vi "Main.vi"() -> ()   [LabVIEW 2017]
doc: "The boiler controller allows a user to start and shut down a boiler.\nUse the Reset, start and Light pilot to sequencially Start the boiler.\nUse the fuel control valve to change the flow of fulel into the boiler.\nUse the Stop button to Shut down the boiler.\nTo shut down the system off ar in the event of emergency, use the emergency stop button to stop the application completely."
uses:
  controls/MHL Data.ctl
  controls/MHL UI Data.ctl
  controls/MHL Status.ctl
  controls/MHL References.ctl
  controls/MHL Configuration.ctl
  support/Boiler System Globals.vi
  <vilib>/Utility/error.llb/Error Cluster From Error Code.vi
  <vilib>/ErrorRing/Error Ring.xnode
  support/Message Queue/Message Queue.lvlib
  support/User Event - Stop/User Event - Stop.lvlib
  Controller/Controller.lvlib
  Boiler/Boiler.lvlib
panel:
  out "Forced Draft Fan":bool
  out "Pilot LED":bool caption="Pilot"
  out "Pilot Gas Valve":bool
  out "Primany Fan":bool
  in  "Fuel Control Valve":u32(slide) scale=10.0..75.0
  in  "Initiate Stop":bool
  in  "Shutdown":bool
  in  "Pilot":bool
  in  "Start Sequence":bool
  in  "Reset":bool
  out "Status":string
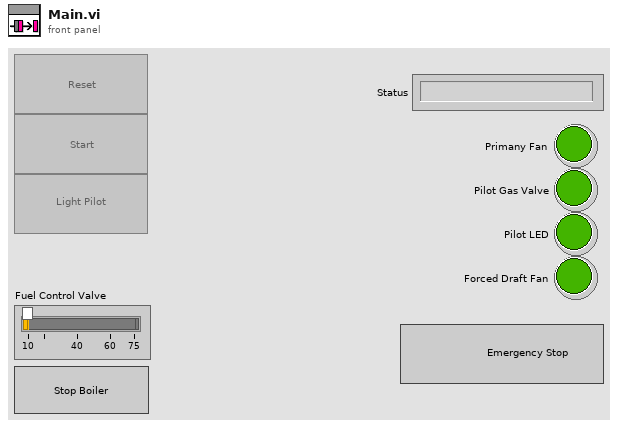
[diagram p1: front panel]
types:
  T1 = typedef "MHL Data.ctl" = cluster{"MHL User Interface Data":T2, "MHL References":T4, "MHL Configuration":T5}
  T2 = typedef "MHL UI Data.ctl" = cluster{"Status":string, "Fuel Control Valve":u32, "Primary Fan":bool, "Pilot Gas Valve":bool, "Pilot":bool, "Forced Draft Fan":bool, "MHL Status":T3}
  T3 = typedef "MHL Status.ctl" = enum16{"Lockout", "Ready", "Pre-Purge", "Pre-Purge Complete", "Pilot On", "Boiler Running", "Shutdown", "Purge"}
  T4 = typedef "MHL References.ctl" = cluster{"Reset Ref":refnum<vi>, "Start Sequence Ref":refnum<vi>, "Pilot Ref":refnum<vi>, "Shutdown Ref":refnum<vi>, "Fuel Control Valve Ref":refnum<vi>}
  T5 = typedef "MHL Configuration.ctl" = cluster{"Fuel Control Valve Maximum":dbl, "Fuel Control Valve Minimum":dbl}
  T6 = typedef "Configuration Data.ctl" = cluster{"MHL Configuration":T5, "Controller Configuration":T7, "Boiler Configuration":T8}
  T7 = typedef "Controller.lvlib/Controller Configuration.ctl" = cluster{"Purge Time":u32, "Flame Threshold":u32}
  T8 = typedef "Boiler.lvlib/Boiler Configuration.ctl" = cluster{"Pilot Increment (ms)":u32, "Pilot Decrement (ms)":u32}
  T9 = typedef "Notifiers.ctl" = cluster{"Handshake":refnum<notifier>, "Flame Level":refnum<notifier>, "Controller Exit":refnum<notifier>, "Boiler Exit":refnum<notifier>}
  T10 = typedef "Message Queue.lvlib/All Message Queues.ctl" = cluster{"MHL":refnum<queue>, "Boiler Controller":refnum<queue>, "Boiler":refnum<queue>}
  T11 = enum16{"open", "replace", "create", "open or create", "replace or create", "replace or create with confirmation"}
  T12 = enum32{"invalid app kind", "Development System", "Run Time System", "Student Edition", "Embedded LabVIEW", "Evaluation", "Custom"}
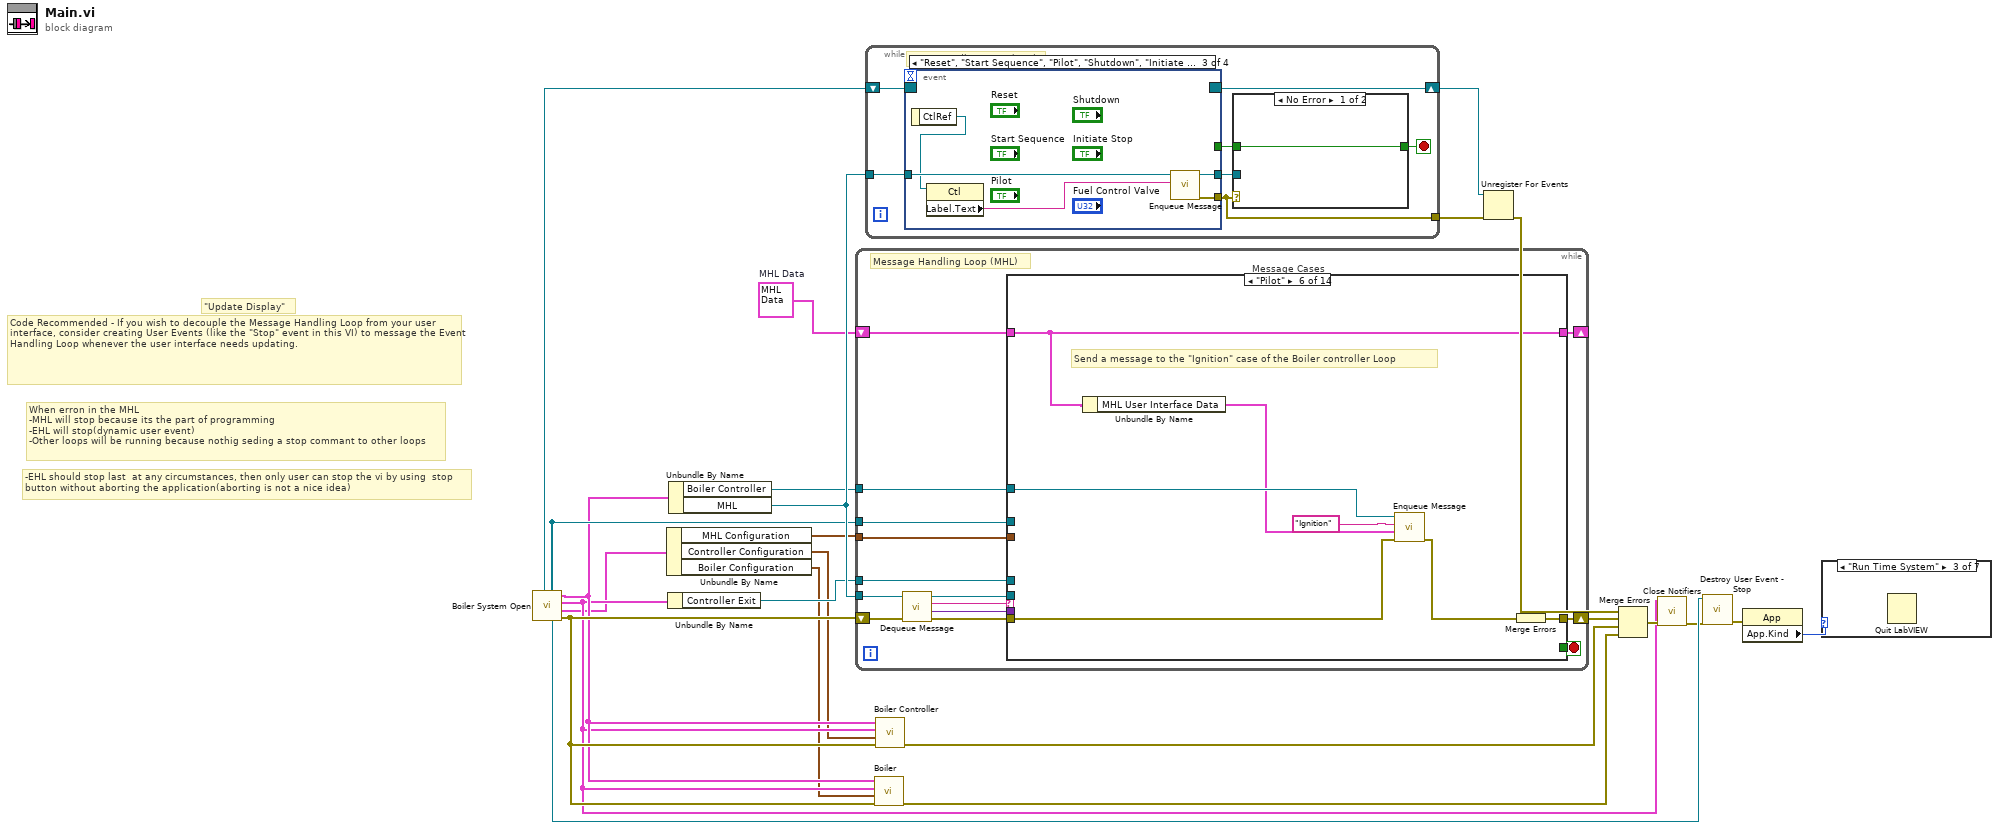
[diagram p0: block diagram]
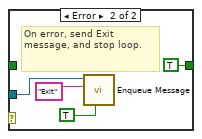
[diagram p8: hidden frame]
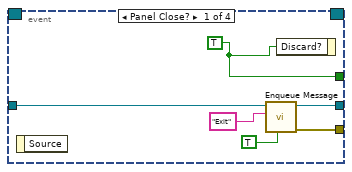
[diagram p9: hidden frame]
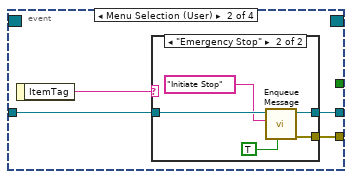
[diagram p10: hidden frame]
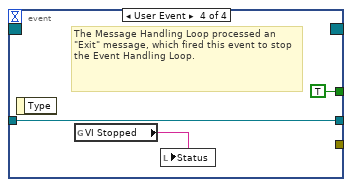
[diagram p12: hidden frame]
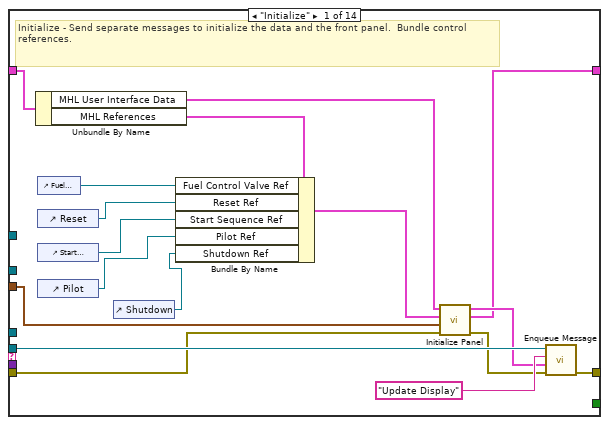
[diagram p13: hidden frame]
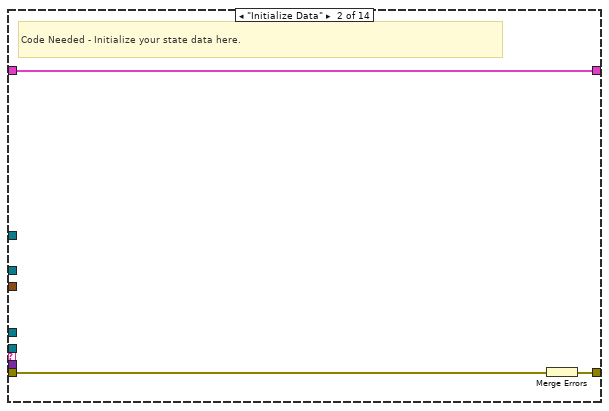
[diagram p14: hidden frame]
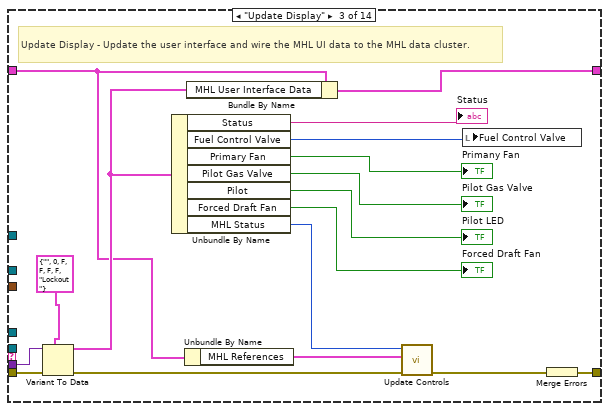
[diagram p15: hidden frame]
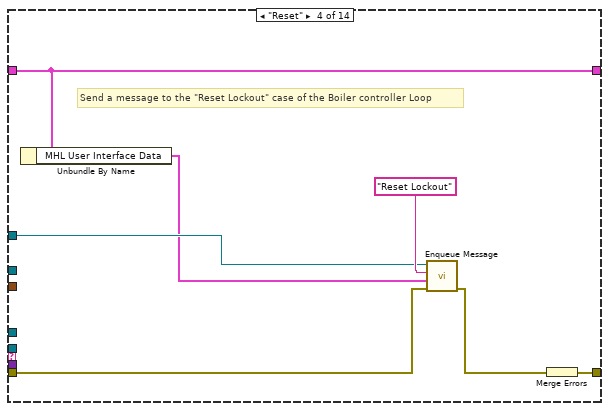
[diagram p16: hidden frame]
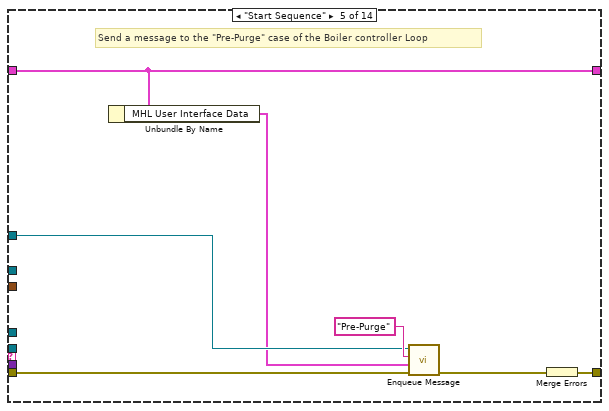
[diagram p17: hidden frame]
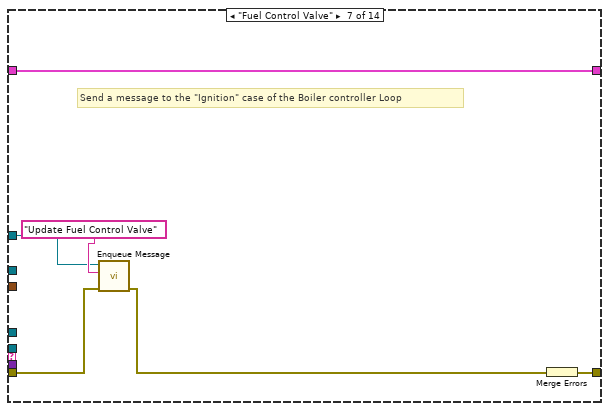
[diagram p18: hidden frame]
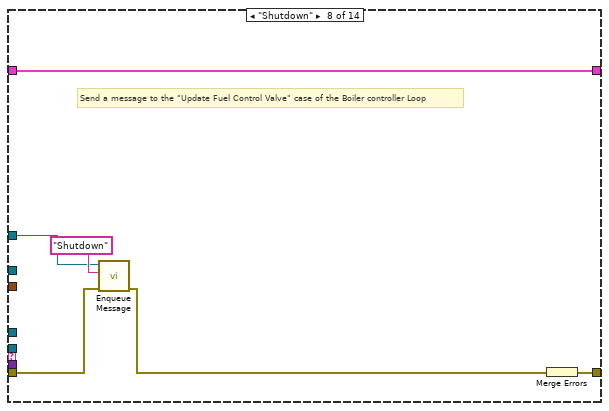
[diagram p19: hidden frame]
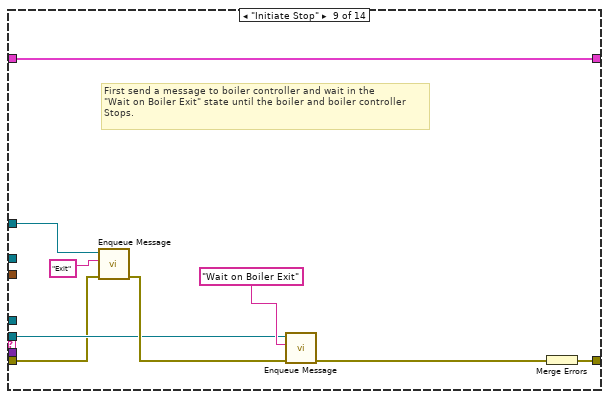
[diagram p20: hidden frame]
diagram:
  w9 = T1 {"MHL User Interface Data"={"Status"="", "Fuel Control Valve"=0, "Primary Fan"=FALSE, "Pilot Gas Valve"=FALSE, "Pilot"=FALSE, "Forced Draft Fan"=FALSE, "MHL Status"=enum."Lockout"}, "MHL References"={"Reset Ref"=refnum, "Start Sequence Ref"=refnum, "Pilot Ref"=refnum, "Shutdown Ref"=refnum, "Fuel Control Valve Ref"=refnum}, "MHL Configuration"={"Fuel Control Valve Maximum"=0.0, "Fuel Control Valve Minimum"=0.0}}  # MHL Data
  # "-EHL should stop last  at any circumstances, then only user can stop the vi by using  stop \nbutton without aborting the application(aborting is not a nice idea)"
  # "When erron in the MHL\n-MHL will stop because its the part of programming\n-EHL will stop(dynamic user event)\n-Other loops will be running because nothig seding a stop commant to other loops"
  # "\"Update Display\""
  # "Code Recommended - If you wish to decouple the Message Handling Loop from your user interface, consider creating User Events (like the \"Stop\" event in this VI) to message the Event Handling Loop whenever the user interface needs updating."
  n1 = call "Boiler System Open.vi"() -> ("error out"=w15:errorcluster, "Configuration Data"=w4:T6, "Notifiers"=w10:T9, "Message Queues out"=w13:T10, "User Event - Stop"=w16:refnum<user-event>, "Stop Event Registration Refnum"=w17:refnum<event-registration>)  [unwired: 6 in]
  n2 = Unbundle By Name(w4) -> ("MHL Configuration"=w3:T5, "Controller Configuration"=w2:T7, "Boiler Configuration"=w1:T8)
  n3 = Unbundle By Name(w10) -> ("Controller Exit"=w14:refnum<notifier>)
  n4 = Unbundle By Name(w13) -> ("Boiler Controller"=w20:refnum<queue>, "MHL"=w21:refnum<queue>)
  n5 = while {
    tunnel: w21 -> [w27]
    shift-right: [w36] -> _
    shift-left: w9 -> [w37]
    tunnel: w16 -> [w33]
    shift-right: [w34] -> w6
    shift-left: w15 -> [w32]
    tunnel: w20 -> [w26]
    tunnel: w14 -> [w25]
    tunnel: w3 -> [w24]
    stop <- w35 stop-if-true
    # "Message Handling Loop (MHL)"
    n6 = call "Dequeue Message.vi"("error in (no error)"=w32, "Message Queue"=w27) -> ("error out"=w31:errorcluster, "Message Data"=w29:variant, "Message"=w30:string, "dup Message Queue"=w28:refnum<queue>)  [unwired: 6 in]
    n7 = case "Message Cases" shown="\"Pilot\"" w30 {
      selector: w30 -> [_ _ _ _ _ _ _ _ _ _ _ _ w170 _]
      tunnel: w28 -> [w51 _ _ _ _ _ _ _ w109 w121 w140 w160 _ _]
      tunnel: w31 -> [w45 w57 w73 w80 w87 w94 w99 w105 w108 w117 w133 w153 _ w181]
      tunnel: [w54 w55 w74 w81 w88 w95 w100 w106 w115 w123 w136 w163 w169 w179] -> w34
      tunnel: w37 -> [w39 w56 w58 w76 w83 w90 w101 w107 w116 w124 w139 w164 w171 w180]
      tunnel: [w38 w56 w69 w76 w83 w90 w101 w107 w116 w124 w139 w164 w171 w180] -> w36
      tunnel: [_ _ _ _ _ _ _ _ _ _ TRUE _ _ _] -> w35
      tunnel: w29 -> [_ _ w72 _ _ _ _ _ _ _ _ w152 _ _]
      tunnel: w33 -> [_ _ _ _ _ _ _ _ _ _ w135 _ _ _]
      tunnel: w26 -> [_ _ _ w77 w84 w91 w96 w102 w110 _ _ _ _ _]
      tunnel: w25 -> [_ _ _ _ _ _ _ _ _ w120 _ _ _ _]
      tunnel: w24 -> [w43 _ _ _ _ _ _ _ _ _ _ _ _ _]
      frame "Initialize" {
        # "Initialize - Send separate messages to initialize the data and the front panel.  Bundle control references."
        n8 = Unbundle By Name(w39) -> ("MHL User Interface Data"=w41:T2, "MHL References"=w52:T4)
        n9 = control-ref of="Fuel Control Valve"() -> (w50:refnum<vi>)
        n10 = control-ref of="Reset"() -> (w49:refnum<vi>)
        n11 = control-ref of="Start Sequence"() -> (w48:refnum<vi>)
        n12 = control-ref of="Pilot"() -> (w47:refnum<vi>)
        n13 = control-ref of="Shutdown"() -> (w46:refnum<vi>)
        n14 = Bundle By Name(cluster=w52, "Fuel Control Valve Ref"=w50, "Reset Ref"=w49, "Start Sequence Ref"=w48, "Pilot Ref"=w47, "Shutdown Ref"=w46) -> (w42:T4)
        n15 = call "Initialize Panel.vi"("error in"=w45, "MHL Configuration"=w43, "MHL References"=w42, "MHL UI Data in"=w41) -> ("error out"=w44:errorcluster, "MHL Data out"=w38:T1, "MHL UI Data out"=w40:T2)  [unwired: 5 in]
        n16 = call "Enqueue Message.vi"("error in (no error)"=w44, "Message Data"=w40, "Message"="Update Display", "Message Queue"=w51) -> ("error out"=w54:errorcluster)  [unwired: 6 in, 1 out]
      }
      frame "Initialize Data" {
        # "Code Needed - Initialize your state data here."
        n17 = Merge Errors(w57) -> (w55:errorcluster)
      }
      frame "Update Display" {
        # "Update Display - Update the user interface and wire the MHL UI data to the MHL data cluster."
        n18 = Variant To Data(error in=w73, type=T2 {"Status"="", "Fuel Control Valve"=0, "Primary Fan"=FALSE, "Pilot Gas Valve"=FALSE, "Pilot"=FALSE, "Forced Draft Fan"=FALSE, "MHL Status"=enum."Lockout"} ("MHL UI Data"), Variant=w72) -> (data=w70:T2, error out=w60:errorcluster)
        n19 = Unbundle By Name(w70) -> ("Status"=→"Status":string, "Fuel Control Valve"=w64:u32, "Primary Fan"=→"Primany Fan":bool, "Pilot Gas Valve"=→"Pilot Gas Valve":bool, "Pilot"=→"Pilot LED":bool, "Forced Draft Fan"=→"Forced Draft Fan":bool, "MHL Status"=w62:T3)
        n20 = Unbundle By Name(w58) -> ("MHL References"=w61:T4)
        n21 = Bundle By Name(cluster=w58, "MHL User Interface Data"=w70) -> (w69:T1)
        n22 = call "Update Controls.vi"("error in"=w60, "MHL References"=w61, "MHL Status"=w62) -> ("error out"=w59:errorcluster)  [unwired: 8 in]
        n23 = local write "Fuel Control Valve"(w64) -> ()
        n24 = Merge Errors(w59) -> (w74:errorcluster)
      }
      frame "Reset" {
        # "Send a message to the \"Reset Lockout\" case of the Boiler controller Loop"
        n25 = Unbundle By Name(w76) -> ("MHL User Interface Data"=w75:T2)
        n26 = call "Enqueue Message.vi"("error in (no error)"=w80, "Message Data"=w75, "Message"="Reset Lockout", "Message Queue"=w77) -> ("error out"=w79:errorcluster)  [unwired: 6 in, 1 out]
        n27 = Merge Errors(w79) -> (w81:errorcluster)
      }
      frame "Start Sequence" {
        # "Send a message to the \"Pre-Purge\" case of the Boiler controller Loop"
        n28 = Unbundle By Name(w83) -> ("MHL User Interface Data"=w82:T2)
        n29 = call "Enqueue Message.vi"("error in (no error)"=w87, "Message Data"=w82, "Message"="Pre-Purge", "Message Queue"=w84) -> ("error out"=w86:errorcluster)  [unwired: 6 in, 1 out]
        n30 = Merge Errors(w86) -> (w88:errorcluster)
      }
      frame "Pilot" {
        # "Send a message to the \"Ignition\" case of the Boiler controller Loop"
        n31 = Unbundle By Name(w90) -> ("MHL User Interface Data"=w89:T2)
        n32 = call "Enqueue Message.vi"("error in (no error)"=w94, "Message Data"=w89, "Message"="Ignition", "Message Queue"=w91) -> ("error out"=w93:errorcluster)  [unwired: 6 in, 1 out]
        n33 = Merge Errors(w93) -> (w95:errorcluster)
      }
      frame "Fuel Control Valve" {
        # "Send a message to the \"Ignition\" case of the Boiler controller Loop"
        n34 = call "Enqueue Message.vi"("error in (no error)"=w99, "Message"="Update Fuel Control Valve", "Message Queue"=w96) -> ("error out"=w98:errorcluster)  [unwired: 7 in, 1 out]
        n35 = Merge Errors(w98) -> (w100:errorcluster)
      }
      frame "Shutdown" {
        # "Send a message to the \"Update Fuel Control Valve\" case of the Boiler controller Loop"
        n36 = call "Enqueue Message.vi"("error in (no error)"=w105, "Message"="Shutdown", "Message Queue"=w102) -> ("error out"=w104:errorcluster)  [unwired: 7 in, 1 out]
        n37 = Merge Errors(w104) -> (w106:errorcluster)
      }
      frame "Initiate Stop" {
        # "First send a message to boiler controller and wait in the \n\"Wait on Boiler Exit\" state until the boiler and boiler controller\nStops."
        n38 = call "Enqueue Message.vi"("error in (no error)"=w108, "Message"="Exit", "Message Queue"=w110) -> ("error out"=w114:errorcluster)  [unwired: 7 in, 1 out]
        n39 = call "Enqueue Message.vi"("error in (no error)"=w114, "Message"="Wait on Boiler Exit", "Message Queue"=w109) -> ("error out"=w113:errorcluster)  [unwired: 7 in, 1 out]
        n40 = Merge Errors(w113) -> (w115:errorcluster)
      }
      frame "Wait on Boiler Exit" {
        # "Monitor the boiler control loop to determine if the boiler loop exit and boiler controller loop \nfinishes its \"Exit\" state.\nWait on notification wait for the notification from boiler controller for  10ms. And if it timed \nout, it continue to stay in the same loop.\nIf MHL gets some notification, it will start its \"exit\" state."
        n41 = Wait on Notification(notifier=w120, timeout in ms (-1)=10) -> (timed out?=w118:bool)  [unwired: 2 in, 3 out]
        n42 = case shown="False" w118 {
          tunnel: [w128 w132] -> w122
          tunnel: w121 -> [w126 w130]
          tunnel: w117 -> [w125 w129]
          frame True {
            n43 = call "Enqueue Message.vi"("Message Data"=w125, "Message"="Wait on Boiler Exit", "Message Queue"=w126) -> ("error out"=w128:errorcluster)  [unwired: 7 in, 1 out]
          }
          frame False {
            n44 = call "Enqueue Message.vi"("error in (no error)"=w129, "Message"="Exit", "Message Queue"=w130) -> ("error out"=w132:errorcluster)  [unwired: 7 in, 1 out]
          }
        }
        n45 = Merge Errors(w122) -> (w123:errorcluster)
      }
      frame "Exit" {
        # "Trigger the dynamic event here"
        # "Stop the VI"
        # "Release the message queue reference"
        # "Code Needed - Add any required cleanup code here"
        n46 = call "Fire User Event - Stop.vi"("User Event - Stop"=w135) -> ("error out"=w134:errorcluster)  [unwired: 10 in]
        n47 = Release Queue(queue=w140, error in (no error)=w133) -> (error out=w137:errorcluster)  [unwired: 1 in, 2 out]
        n48 = Merge Errors(w134, w137) -> (w136:errorcluster)
      }
      frame "Error" {
        # "First send a message to boiler controller and wait in the \n\"Wait on Boiler Exit\" state until the boiler and boiler controller\nStops."
        n49 = Variant To Data(error in=w153, type=errorcluster {"status"=FALSE, "code"=0, "source"=""} ("error constant"), Variant=w152) -> (data=w149:errorcluster, error out=w150:errorcluster)
        n50 = call <vilib>:"Application Directory.vi"() -> ("Application Directory"=w159:path)
        n51 = Merge Errors(w149, w150) -> (w148:errorcluster)
        n52 = Build Path(base path=w159, name or relative path=path "Log Error.txt") -> (appended path=w157:path)
        n53 = Unbundle By Name(w148) -> ("code"=w147:i32, "source"=w146:string)
        n54 = Open/Create/Replace File(file path (use dialog)=w157, operation (0:open)=T11."open or create") -> (refnum out=w154:refnum<file>, error out=w155:errorcluster)  [unwired: 4 in, 1 out]
        n55 = call <vilib>:"Clear Errors.vi"("error in (no error)"=w155) -> ("error out"=w145:errorcluster)  [unwired: 5 in, 1 out]
        n56 = call "Log Error.vi"("error in"=w145, "Source"=w146, "Code"=w147, "Error Log Refnum In"=w154) -> ("error out"=w142:errorcluster, "Error Log Refnum Out"=w143:refnum<file>)  [unwired: 6 in]
        n57 = Not A Number/Path/Refnum?(number/path/refnum=w143) -> (NaN/Path/Refnum?=w144:bool)
        n58 = case shown="False" w144 {
          tunnel: w143 -> [w165 _]
          tunnel: w142 -> [w167 w168]
          tunnel: [w166 w168] -> w141
          frame False {
            n59 = Close File(refnum=w165, error in=w167) -> (error out=w166:errorcluster)  [unwired: 1 out]
          }
          frame True {
          }
        }
        n60 = call "Enqueue Message.vi"("error in (no error)"=w141, "Message"="Initiate Stop", "Message Queue"=w160) -> ("error out"=w162:errorcluster)  [unwired: 7 in, 1 out]
        n61 = Merge Errors(w162) -> (w163:errorcluster)
      }
      frame Default {
        # "'Default' case only runs if there is a message that isn't defined in any of the other cases.  Output a programming error."
        n62 = xnode "Error Ring"("parameter 0"=w170) -> ("error out"=w169:errorcluster)
      }
      frame "---Copy This Frame---" {
        # "Duplicate this frame when creating new messages.  Change this comment in the duplicated frame to describe this message."
        n63 = Merge Errors(w181) -> (w179:errorcluster)
      }
    }
  }
  n64 = while {
    tunnel: w21 -> [w188]
    tunnel: [w184] -> w5
    shift-right: [w182] -> w22
    shift-left: w17 -> [w183]
    stop <- w186 stop-if-true
    # "Event Handling Loop (EHL)"
    n65 = event shown="[2] \"Reset\", \"Start Sequence\", \"Pilot\", \"Shutdown\", \"Initiate Stop\", \"Fuel Control Valve\": Value Change" {
      selector: w183 -> [_ _ _ _]
      dyn-events: [_ _ _ _] -> w182
      timeout: _ -> [_ _ _ _]
      tunnel: [w194 _ _ TRUE ("Discard?")] -> w187
      tunnel: w188 -> [w199 w203 w214 w217]
      tunnel: [w198 w202 w213 _] -> w184
      tunnel: [w197 w201 w212 w217] -> w185
      event Panel Close? {
        w194 = TRUE ("Discard?")
        n66 = event-data() -> ()  [unwired: 1 in, 1 out]
        n67 = call "Enqueue Message.vi"("Priority Message? (F)"=TRUE, "Message"="Exit", "Message Queue"=w199) -> ("error out"=w198:errorcluster, "dup Message Queue"=w197:refnum<queue>)  [unwired: 7 in]
        n68 = event-data("Discard?"=w194) -> ()  [unwired: 1 in, 1 out]
      }
      event Menu Selection (User) {
        n69 = event-data() -> ("ItemTag"=w200:string)  [unwired: 1 in]
        n70 = case shown="\"Emergency Stop\"" w200 {
          tunnel: w203 -> [w204 w209]
          tunnel: [_ w208] -> w202
          tunnel: [w204 w207] -> w201
          frame Default {
          }
          frame "Emergency Stop" {
            n71 = call "Enqueue Message.vi"("Priority Message? (F)"=TRUE, "Message"="Initiate Stop", "Message Queue"=w209) -> ("error out"=w208:errorcluster, "dup Message Queue"=w207:refnum<queue>)  [unwired: 7 in]
          }
        }
      }
      event "Reset", "Start Sequence", "Pilot", "Shutdown", "Initiate Stop", "Fuel Control Valve": Value Change {
        n72 = event-data() -> ("CtlRef"=w211:refnum<vi>)  [unwired: 1 in]
        n73 = property class="Ctl"(reference=w211) -> ("Label.Text"=w210:string)  [unwired: 1 in, 2 out]
        n74 = call "Enqueue Message.vi"("Message"=w210, "Message Queue"=w214) -> ("error out"=w213:errorcluster, "dup Message Queue"=w212:refnum<queue>)  [unwired: 8 in]
      }
      event User Event {
        # "The Message Handling Loop processed an \"Exit\" message, which fired this event to stop the Event Handling Loop."
        n75 = event-data() -> ()  [unwired: 1 in, 1 out]
        n76 = global read "Boiler System Globals.vi" "VI Stopped"() -> (w215:string)
        n77 = local write "Status"(w215) -> ()
      }
    }
    n78 = case shown="No Error" w184 {
      tunnel: [w189 TRUE ("Discard?")] -> w186
      tunnel: w187 -> [w189 _]
      tunnel: w185 -> [_ w192]
      frame No Error {
      }
      frame Error {
        # "On error, send Exit message, and stop loop."
        n79 = call "Enqueue Message.vi"("Priority Message? (F)"=TRUE, "Message"="Exit", "Message Queue"=w192) -> ()  [unwired: 7 in, 2 out]
      }
    }
  }
  n80 = call "Boiler.vi"("error in"=w15, "Boiler Configuration"=w1, "Notifiers"=w10, "Message Queues"=w13) -> ("error out"=w7:errorcluster)  [unwired: 7 in]
  n81 = call "Boiler Controller.vi"("error in (no error)"=w15, "Controller Configuration Data"=w2, "Notifiers"=w10, "All Message Queues"=w13) -> ("error out"=w8:errorcluster)  [unwired: 7 in]
  n82 = Unregister For Events(event registration refnum=w22, error in=w5) -> (error out=w23:errorcluster)
  n83 = Merge Errors(w23, w6, w8, w7) -> (w12:errorcluster)
  n84 = call "Close Notifiers.vi"("error constant"=w12, "output cluster"=w10) -> ("error out"=w11:errorcluster)  [unwired: 9 in]
  n85 = call "Destroy User Event - Stop.vi"("error in (no error)"=w11, "User Event - Stop"=w16) -> ("error out"=w19:errorcluster)  [unwired: 9 in]
  n86 = property class="App"(error in=w19) -> ("App.Kind"=w18:T12)  [unwired: 1 in, 2 out]
  n87 = case shown="\"Run Time System\"" w18 {
    frame "invalid app kind", Default {
    }
    frame "Development System" {
    }
    frame "Run Time System" {
      n88 = Quit LabVIEW() -> ()  [unwired: 1 in]
    }
    frame "Student Edition" {
    }
    frame "Embedded LabVIEW" {
    }
    frame "Evaluation" {
    }
    frame "Custom" {
    }
  }
